vi "Report display.vi"(8 "error in (no error)":errorcluster, 11 "Tomo in":refnum<class "Tomo.lvclass">) -> (0 "error out":errorcluster, 3 "Tomo out":refnum<class "Tomo.lvclass">)   [LabVIEW 2012, in "Tomo.lvclass"]
uses:
  Tomo.lvclass
  Tomo.lvclass/Tomo.ctl
panel:
  out "last stack time":timestamp
  out "experimenter name":string
  out "experiment name":string
  out "z_stop":dbl
  out "z_start":dbl
  out "y":dbl
  out "x":dbl
  out "total stacks":u16
  out "current stack":u16
  # "Tomography"
  # "started by"
  # "Currently acquiring stack"
  # "of"
  # "last stack acquired at"
  # "Coordinates"
  # "x"
  # "y"
  # "z start"
  # "z stop"
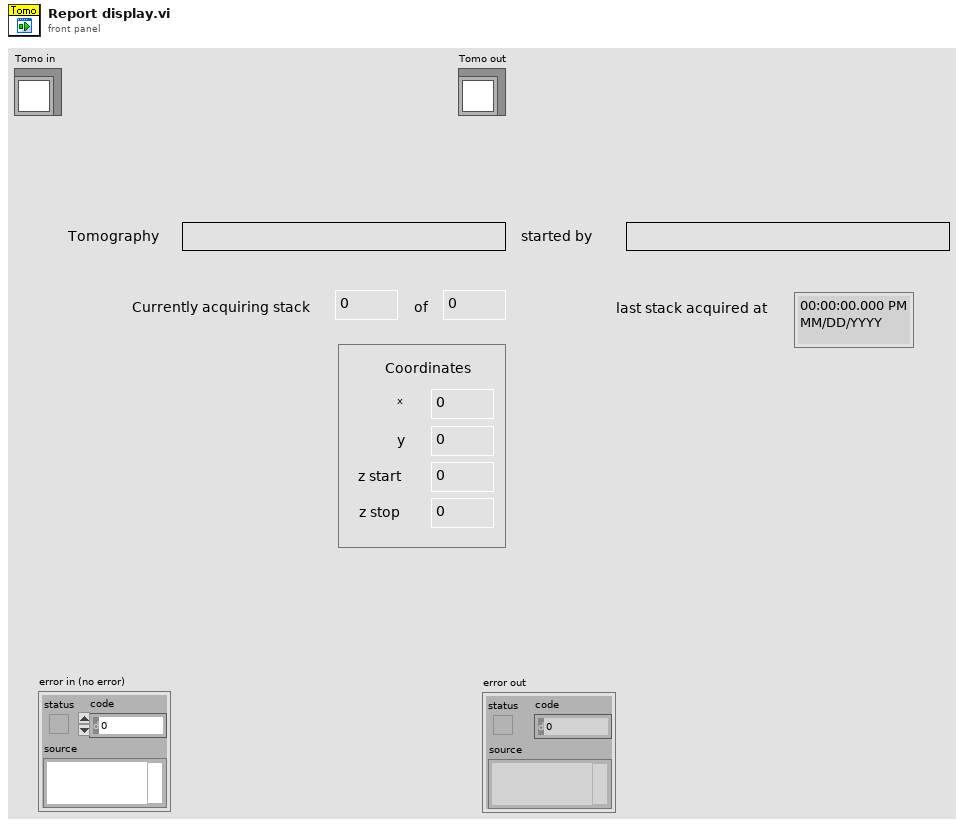
[diagram p1: front panel]
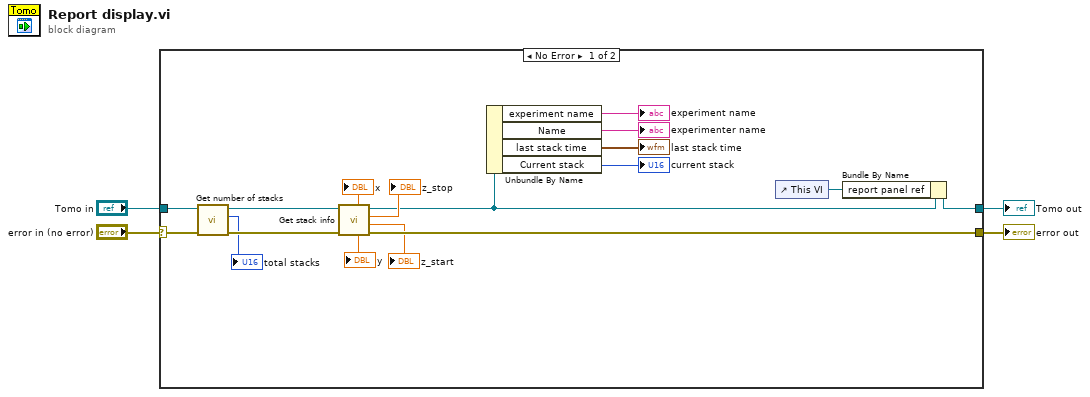
[diagram p0: block diagram]
diagram:
  n1 = case shown="No Error" "error in (no error)" {
    selector: "error in (no error)" -> [w18 w23]
    tunnel: [w16 w23] -> w3
    tunnel: [w6 w22] -> w1
    tunnel: "Tomo in" -> [w20 w22]
    frame No Error {
      n2 = call-dynamic "Get number of stacks.vi"("error in (no error)"=w18, "Tomo in"=w20) -> ("error out"=w17:errorcluster, "Number of stacks"=→"total stacks":u16, "Tomo out"=w19:refnum<class "Tomo.lvclass">)  [unwired: 7 in]
      n3 = call-dynamic "Get stack info.vi"("error in (no error)"=w17, "Tomo in"=w19) -> ("error out"=w16:errorcluster, "Z start"=→"z_start":dbl, "Z stop"=→"z_stop":dbl, "Tomo out"=w7:refnum<class "Tomo.lvclass">, "Y position"=→"y":dbl, "X position"=→"x":dbl)  [unwired: 4 in]
      n4 = Unbundle By Name(w7) -> ("experiment name"=→"experiment name":string, "Name"=→"experimenter name":string, "last stack time"=→"last stack time":timestamp, "Current stack"=→"current stack":u16)
      n5 = control-ref of="This VI"() -> (w5:refnum<vi>)
      n6 = Bundle By Name(cluster=w7, "report panel ref"=w5) -> (w6:refnum<class "Tomo.lvclass">)
    }
    frame Error {
    }
  }
  "error out" <- w3
  "Tomo out" <- w1
